vi "Turn F Immediatly But Ture T with Latency.vi"(7 "Reset(F)":bool, 8 "计时时长(ms)":u32=5000, 11 "Signal":bool) -> (0 "变化过去时间(ms)":u32, 3 "signal(safe)":bool)   [LabVIEW 2017]
doc: "Follows Signal, turning the output FALSE immediately but delaying the transition to TRUE by the timing duration (ms)."
uses:
  5093cefc-d3d2-4eb3-bc00-370220dfee7f.vi
  d8dc2e1a-5964-4f74-9887-ef2f57e1a81f.vi
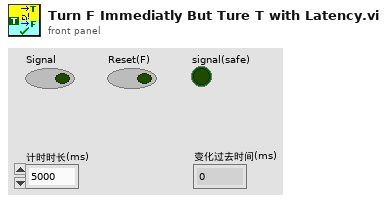
[diagram p1: front panel]
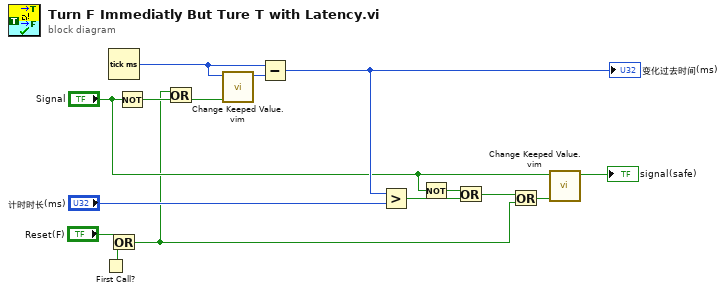
[diagram p0: block diagram]
diagram:
  n1 = First Call?() -> (First Call?: T/F=w6:bool)
  n2 = Tick Count (ms)() -> (millisecond timer value=w14:u32)
  n3 = Or(x="Reset(F)", y=w6) -> (x .or. y?=w1:bool)
  n4 = Not(x="Signal") -> (.not. x?=w8:bool)
  n5 = Or(x=w1, y=w8) -> (x .or. y?=w2:bool)
  n6 = call "Change Keeped Value.vim"("change?"=w2, "new value"=w14) -> ("keeped value"=w15:u32)  [unwired: 9 in]
  n7 = Subtract(x=w14, y=w15) -> (x-y=w10:u32)
  "变化过去时间(ms)" <- w10
  n8 = Greater?(x=w10, y="计时时长(ms)") -> (0:w11:bool)
  n9 = Not(x="Signal") -> (.not. x?=w12:bool)
  n10 = Or(x=w12, y=w11) -> (x .or. y?=w7:bool)
  n11 = Or(x=w7, y=w1) -> (x .or. y?=w4:bool)
  n12 = call "Change Keeped Value.vim"("change?"=w4, "new value"="Signal") -> ("keeped value"=→"signal(safe)":bool)  [unwired: 9 in]
